vi "Initialize.vi"(8 "error in":errorcluster, 10 "resource name":T1, 11 "lia rt in":refnum<class "Lock-In Amplifier Example RT.lvclass">) -> (0 "error out":errorcluster, 3 "lia rt out":refnum<class "Lock-In Amplifier Example RT.lvclass">)   [LabVIEW 2017, in "Lock-In Amplifier Example RT.lvclass"]
uses:
  Lock-In Amplifier Example RT.lvclass
  <vilib>/userdefined/High Color/nirio_resource_hc.ctl
  Private/session data.ctl
  server/RT FlexRIO Server TCP.lvclass
  interface/Interface FPGA/LIA Host Interface FPGA.lvclass
  Lock-In Amplifier Example RT.lvclass/Lock-In Amplifier Example RT.ctl
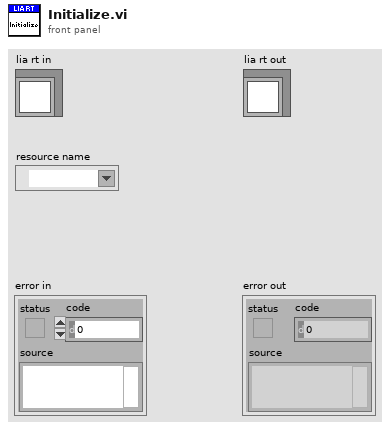
[diagram p1: front panel]
types:
  T1 = typedef "nirio_resource_hc.ctl" = tag
  T2 = typedef "Lock-In Amplifier Example RT.lvclass/session data.ctl" = cluster{"server":refnum<class "RT FlexRIO Server TCP.lvclass">, "fpga interface":refnum<class "LIA Host Interface FPGA.lvclass">}
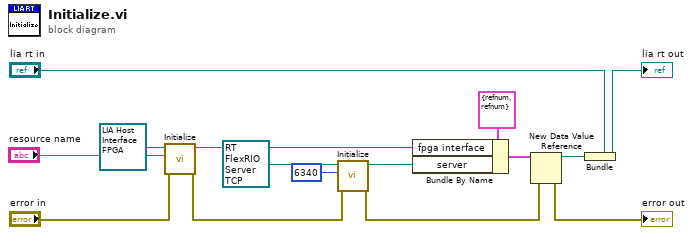
[diagram p0: block diagram]
diagram:
  n1 = call-dynamic "Initialize.vi"("error in"="error in", "resource"="resource name", "host in"=refnum<class "LIA Host Interface FPGA.lvclass"> refnum ("lia host")) -> ("error out"=w3:errorcluster, "host out"=w4:refnum<class "LIA Host Interface FPGA.lvclass">)  [unwired: 7 in]
  n2 = call-dynamic "Initialize.vi"("error in"=w3, "port"=u16 6340, "server in"=refnum<class "RT FlexRIO Server TCP.lvclass"> refnum ("tcp server in")) -> ("error out"=w9:errorcluster, "server in"=w8:refnum<class "RT FlexRIO Server TCP.lvclass">)  [unwired: 7 in]
  n3 = Bundle By Name(cluster=T2 {"server"=refnum, "fpga interface"=refnum} ("Cluster"), "fpga interface"=w4, "server"=w8) -> (w14:T2)
  n4 = New Data Value Reference(data value=w14, error in=w9) -> (data value reference=w13:refnum<data-value>, error out=→"error out":errorcluster)
  n5 = Bundle(cluster="lia rt in", w13) -> (→"lia rt out":refnum<class "Lock-In Amplifier Example RT.lvclass">)
